vi "HW_GEN - Search for Modu CFG according to Tag.vi"(10 "ModuTag":string, 11 "ModuCFG[]":T1[](array[typedef])) -> (2 "find?":bool, 3 "ModuCFG out":T1, 5 "idx":i32)   [LabVIEW 2016]
uses:
  Ctrls/HardWare _ Module Configuration.ctl
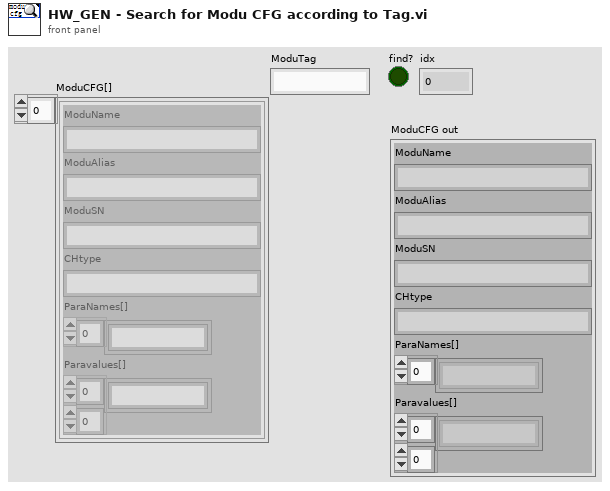
[diagram p1: front panel]
types:
  T1 = typedef "HardWare _ Module Configuration.ctl" = cluster{"ModuName":string, "ModuAlias":string, "ModuSN":string, "CHtype":string, "ParaNames[]":string[], "Paravalues[]":string[][]}
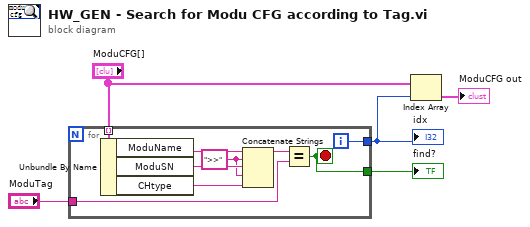
[diagram p0: block diagram]
diagram:
  n1 = for {
    tunnel: "ModuTag" -> [w14]
    tunnel: [w12] -> w4
    tunnel: "ModuCFG[]" -> [w7] mode=indexing
    tunnel: [w6] -> w2
    i -> [w6]
    stop <- w12 stop-if-true
    w8 = ">>" ("string")
    n2 = Unbundle By Name(w7) -> ("ModuName"=w13:string, "ModuSN"=w10:string, "CHtype"=w9:string)
    n3 = Concatenate Strings(w13, w8, w10, w8, w9) -> (w11:string)
    n4 = Equal?(x=w11, y=w14) -> (x = y?=w12:bool)
  }
  "find?" <- w4
  "idx" <- w2
  n5 = Index Array(array="ModuCFG[]", index=w2) -> (element=→"ModuCFG out":T1)
